vi "RT-test.vi"(8 "RT_Input":T7={"Load"=FALSE, "History_[CAD]"=63, "Stall_Speed_[RPM]"=200.0} caption="簇", 9 "EPTxState":T5, 10 "Filters (0)":T6 {"Aux_4_[s]" format="%#_6p"; "Aux_3_[s]" format="%#_6p"; "Aux_2_[s]" format="%#_6p"; "Aux_1_[s]" format="%#_6p"; "Primary_[s]" format="%#_6p"}, 11 "布尔":bool) -> (0 "Loading":bool, 1 "EPTxControl":T2={"Sync_Enable"=FALSE, "Clear_Errors"=FALSE, "Sim_Enable"=FALSE, "Sim_Rate"=63.999996185302734, "Watchdog"=FALSE}, 2 "EPTxConfig":T3, 3 "Max CAD":sgl=63.0 format="%.2f", 4 "布尔 2":bool)   [LabVIEW 2020]
uses:
  <vilib>/Powertrain Controls/Device Drivers/Engine Position Tracking/EPTx/RevA/RT/Controls/EPTxFilters.ctl
  <vilib>/Powertrain Controls/Device Drivers/Engine Position Tracking/EPTx/RevA/RT/Controls/EPTxState.ctl
  <vilib>/Powertrain Controls/Device Drivers/Engine Position Tracking/EPTx/RevA/FPGA/Controls/EPTxSupervisor.ctl
  <vilib>/Powertrain Controls/Device Drivers/Engine Position Tracking/EPTx/RevA/FPGA/Controls/EPTxConfig.ctl
  <vilib>/Powertrain Controls/Device Drivers/Engine Position Tracking/EPTx/RevA/FPGA/Controls/EPTxControl.ctl
  <vilib>/Powertrain Controls/Device Drivers/Engine Position Tracking/EPTx/RevA/RT/Controls/EPTxData.ctl
  <vilib>/Powertrain Controls/Device Drivers/Engine Position Tracking/EPTx/RevA/RT/Controls/EPTxSettings.ctl
  <vilib>/Powertrain Controls/Device Drivers/Engine Position Tracking/EPTx/RevA/RT/Controls/Settings - Tooth.ctl
  <vilib>/Powertrain Controls/Device Drivers/Engine Position Tracking/EPTx/RevA/RT/Controls/Direction Detection.ctl
  <vilib>/Powertrain Controls/Device Drivers/Engine Position Tracking/EPTx/RevA/RT/Controls/Settings - Pattern.ctl
  <vilib>/Powertrain Controls/Device Drivers/Engine Position Tracking/EPTx/RevA/RT/Controls/Settings - Token.ctl
  <vilib>/Powertrain Controls/Device Drivers/Engine Position Tracking/EPTx/RevA/RT/Controls/Aux Signal.ctl
  <vilib>/Powertrain Controls/Device Drivers/Engine Position Tracking/EPTx/RevA/RT/Controls/Aux Type.ctl
  <vilib>/Powertrain Controls/Device Drivers/Engine Position Tracking/EPTx/RevA/RT/Controls/Aux Threshold.ctl
  <vilib>/Powertrain Controls/Device Drivers/Engine Position Tracking/EPTx/RevA/RT/EPTx - RevA - RT.lvlib
  <vilib>/Powertrain Controls/Device Drivers/Engine Position Tracking/EPTx/RevA/FPGA/EPTx - RevA - FPGA.lvlib
panel:
  out "EPTxData":T1
  in  "EPTxSupervisor":T4={"Sync"=FALSE, "CurrentCAD"=0.0, "MaxCAD"=720.0, "HistoryCAD"=61.0, "CADRate"=0.0, "AvgSpeed"=0.0, "Config"=FALSE, "Rcvg_Primary"=FALSE, "Stall"=FALSE, "Overflow"=FALSE, "Ratio_Error"=FALSE, "Pattern_Error"=FALSE, "Aux_Warning"=FALSE, "Watchdog_Error"=FALSE}
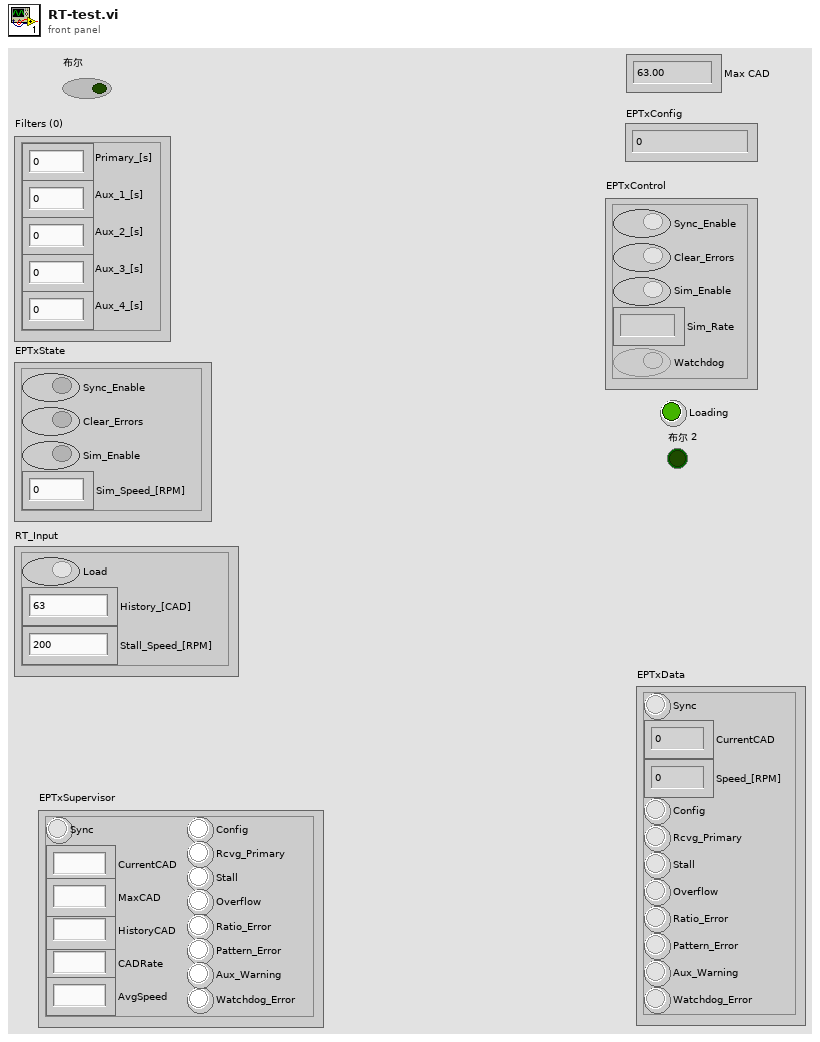
[diagram p1: front panel]
types:
  T1 = typedef "EPTx - RevA - RT.lvlib/EPTxData.ctl" = cluster{"Sync":bool, "CurrentCAD":sgl, "Speed_[RPM]":sgl, "Config":bool, "Rcvg_Primary":bool, "Stall":bool, "Overflow":bool, "Ratio_Error":bool, "Pattern_Error":bool, "Aux_Warning":bool, "Watchdog_Error":bool}
  T2 = typedef "EPTx - RevA - FPGA.lvlib/EPTxControl.ctl" = cluster{"Sync_Enable":bool, "Clear_Errors":bool, "Sim_Enable":bool, "Sim_Rate":fxp<+,24,6>, "Watchdog":bool}
  T3 = typedef "EPTx - RevA - FPGA.lvlib/EPTxConfig.ctl" = u64
  T4 = typedef "EPTx - RevA - FPGA.lvlib/EPTxSupervisor.ctl" = cluster{"Sync":bool, "CurrentCAD":fxp<+,18,11>, "MaxCAD":fxp<+,11,11>, "HistoryCAD":fxp<+,11,11>, "CADRate":fxp<+,22,8>, "AvgSpeed":fxp<+,17,15>, "Config":bool, "Rcvg_Primary":bool, "Stall":bool, "Overflow":bool, "Ratio_Error":bool, "Pattern_Error":bool, "Aux_Warning":bool, "Watchdog_Error":bool}
  T5 = typedef "EPTx - RevA - RT.lvlib/EPTxState.ctl" = cluster{"Sync_Enable":bool, "Clear_Errors":bool, "Sim_Enable":bool, "Sim_Speed_[RPM]":sgl}
  T6 = typedef "EPTx - RevA - RT.lvlib/EPTxFilters.ctl" = cluster{"Primary_[s]":sgl, "Aux_1_[s]":sgl, "Aux_2_[s]":sgl, "Aux_3_[s]":sgl, "Aux_4_[s]":sgl}
  T7 = cluster{"Load":bool, "History_[CAD]":u8, "Stall_Speed_[RPM]":sgl}
  T8 = typedef "EPTx - RevA - RT.lvlib/EPTxSettings.ctl" = cluster{"Rotation":u8, "Ratios":sgl[], "Thresholds":sgl[], "Tooth":T9, "Pattern":T11[], "Token":T12[], "Aux Threshold Min":T15, "Aux Threshold Max":T15}
  T9 = typedef "EPTx - RevA - RT.lvlib/Settings - Tooth.ctl" = cluster{"Rising Edge":bool, "Falling Edge":bool, "Direction\nDetection":T10, "Level":bool, "Parameter":sgl}
  T10 = typedef "EPTx - RevA - RT.lvlib/Direction Detection.ctl" = enum16{"None", "Aux Signal", "Length"}
  T11 = typedef "EPTx - RevA - RT.lvlib/Settings - Pattern.ctl" = cluster{"Ratio Index":u8, "Ratio Count":u16, "Angle":sgl, "dAngle":sgl}
  T12 = typedef "EPTx - RevA - RT.lvlib/Settings - Token.ctl" = cluster{"Length":u16, "Start Index":u8, "Start Count":u16, "Aux 1":T13, "Aux 1 Type":T14, "Aux 1 Max":u16, "Aux 1 Min":u16, "Aux 2":T13, "Aux 2 Type":T14, "Aux 2 Max":u16, "Aux 2 Min":u16, "End Index":u8, "End Count":u16}
  T13 = typedef "EPTx - RevA - RT.lvlib/Aux Signal.ctl" = enum8{"---", "Aux 1", "Aux 2", "Aux 3", "Aux 4"}
  T14 = typedef "EPTx - RevA - RT.lvlib/Aux Type.ctl" = enum8{"Falling", "Rising", "Low", "High", "Ratio"}
  T15 = typedef "EPTx - RevA - RT.lvlib/Aux Threshold.ctl" = cluster{"Aux 1":sgl, "Aux 2":sgl, "Aux 3":sgl, "Aux 4":sgl}
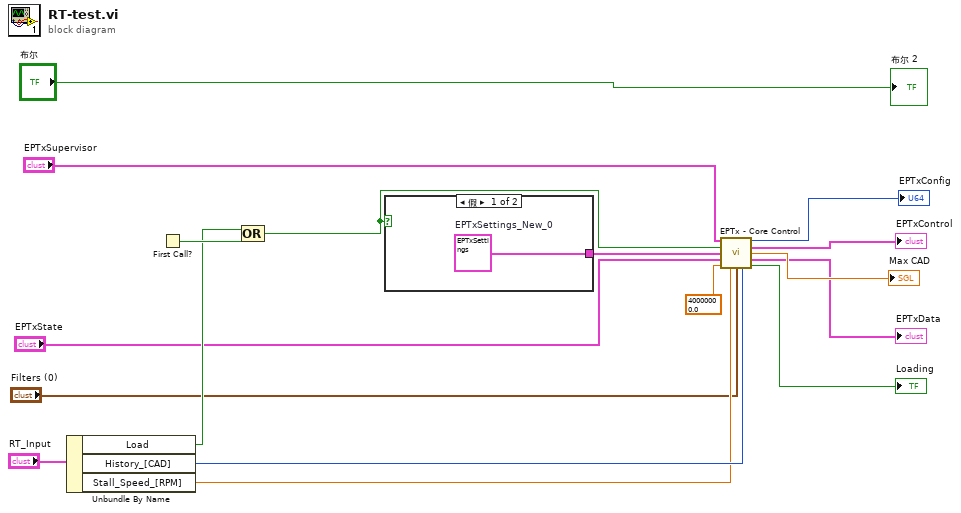
[diagram p0: block diagram]
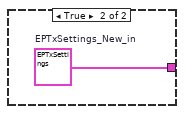
[diagram p2: hidden frame]
diagram:
  n1 = Unbundle By Name("RT_Input") -> ("Load"=w13:bool, "History_[CAD]"=w12:u8, "Stall_Speed_[RPM]"=w11:sgl)
  n2 = First Call?() -> (First Call?: T/F=w15:bool)
  n3 = Compound Arithmetic op=OR ("复合运算")(w13, w15) -> (w9:bool)
  n4 = case shown="假" w9 {
    tunnel: [w18 w19] -> w16
    frame False {
      w18 = T8 {"Rotation"=0, "Ratios"=[], "Thresholds"=[], "Tooth"={"Rising Edge"=FALSE, "Falling Edge"=FALSE, "Direction\nDetection"=enum."None", "Level"=FALSE, "Parameter"=0.0}, "Pattern"=[], "Token"=[], "Aux Threshold Min"={"Aux 1"=0.0, "Aux 2"=0.0, "Aux 3"=0.0, "Aux 4"=0.0}, "Aux Threshold Max"={"Aux 1"=0.0, "Aux 2"=0.0, "Aux 3"=0.0, "Aux 4"=0.0}}  # EPTxSettings_New_0
    }
    frame True {
      w19 = T8 {"Rotation"=2, "Ratios"=[0.33333334, 1.0, 3.0], "Thresholds"=[0.16666667, 0.6666667, 0.6666667, 2.0, 2.0, 4.0, 999.0], "Tooth"={"Rising Edge"=TRUE, "Falling Edge"=FALSE, "Direction\nDetection"=enum."None", "Level"=FALSE, "Parameter"=0.0}, "Pattern"=[{"Ratio Index"=0, "Ratio Count"=1, "Angle"=0.0, "dAngle"=6.0}, {"Ratio Index"=1, "Ratio Count"=56, "Angle"=6.0, "dAngle"=6.0}, {"Ratio Index"=2, "Ratio Count"=1, "Angle"=342.0, "dAngle"=18.0}, {"Ratio Index"=0, "Ratio Count"=1, "Angle"=360.0, "dAngle"=6.0}, {"Ratio Index"=1, "Ratio Count"=56, "Angle"=366.0, "dAngle"=6.0}, {"Ratio Index"=2, "Ratio Count"=1, "Angle"=702.0, "dAngle"=18.0}], "Token"=[{"Length"=1, "Start Index"=5, "Start Count"=0, "Aux 1"=enum."---", "Aux 1 Type"=enum."Falling", "Aux 1 Max"=0, "Aux 1 Min"=0, "Aux 2"=enum."Aux 2", "Aux 2 Type"=enum."Ratio", "Aux 2 Max"=73, "Aux 2 Min"=73, "End Index"=0, "End Count"=0}], "Aux Threshold Min"={"Aux 1"=1.8809524, "Aux 2"=1.2142857, "Aux 3"=0.0, "Aux 4"=0.0}, "Aux Threshold Max"={"Aux 1"=2.7857144, "Aux 2"=1.8809524, "Aux 3"=999.0, "Aux 4"=999.0}}  # EPTxSettings_New_in
    }
  }
  n5 = call <vilib>:"EPTx - Core Control.vi"("EPTxSupervisor"="EPTxSupervisor", "Load"=w9, "EPTxSettings"=w16, "EPTxState"="EPTxState", "Frequency (40M) [Hz]"=sgl 40000000.0, "Stall Speed (200) [RPM]"=w11, "Filters (0)"="Filters (0)", "History (63) [CAD]"=w12) -> ("EPTxConfig"=→"EPTxConfig":T3, "EPTxControl"=→"EPTxControl":T2, "Max CAD"=→"Max CAD":sgl, "EPTxData"=→"EPTxData":T1, "Loading"=→"Loading":bool)  [unwired: 3 in]
  "布尔 2" <- "布尔"
